vi "SaveasPython.vi"(11 "Graph in":refnum<vi>) -> ()   [LabVIEW 2022 SP3]
uses:
  <vilib>/Utility/error.llb/Trim Whitespace One-Sided.vi
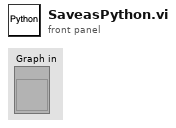
[diagram p1: front panel]
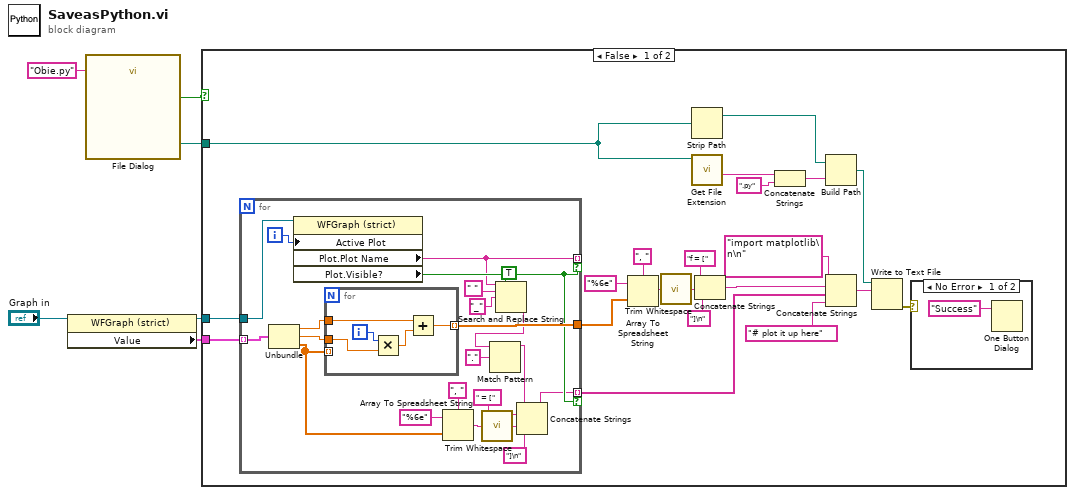
[diagram p0: block diagram]
diagram:
  n1 = property on="Property Node" class="WFGraph (strict)"(reference="Graph in") -> (reference out=w6:refnum<vi>, "Value"=w5:cluster{"x0":dbl, "df":dbl, dbl[]}[])  [unwired: 1 in, 1 out]
  n2 = call "File Dialog"("default name"="Obie.py") -> ("selected path"=w3:path, "cancelled"=w2:bool)  [unwired: 11 in, 2 out]
  n3 = case shown="False" w2 {
    tunnel: w6 -> [w23 _]
    tunnel: w5 -> [w22 _]
    tunnel: w3 -> [w21 _]
    frame False {
      n4 = for {
        tunnel: [w48] -> w13
        tunnel: w22 -> [w47] mode=indexing
        tunnel: [w38] -> w10 mode=indexing if=w44
        tunnel: [w35] -> _ mode=indexing if=w44
        tunnel: w23 -> [w46]
        i -> [w45]
        n5 = Unbundle(w47) -> ("x0"=w49:dbl, "df"=w50:dbl, w42:dbl[])
        n6 = property on="Property Node" class="WFGraph (strict)"(reference=w46, "Active Plot"=w45) -> ("Plot.Plot Name"=w35:string, "Plot.Visible?"=w44:bool)  [unwired: 1 in, 2 out]
        n7 = for {
          tunnel: w50 -> [w54]
          tunnel: w49 -> [w52]
          tunnel: [w51] -> w48 mode=indexing
          tunnel: w42 -> [_] mode=indexing
          i -> [w53]
          n8 = Multiply(x=w53, y=w54) -> (x*y=w55:dbl)
          n9 = Add(x=w52, y=w55) -> (x+y=w51:dbl)
        }
        n10 = Array To Spreadsheet String(delimiter (Tab)=", ", array=w42, 3:"%6e" ("format string")) -> (spreadsheet string=w40:string)
        n11 = call <vilib>:"Trim Whitespace.vi"("string"=w40) -> ("trimmed string"=w36:string)  [unwired: 1 in]
        n12 = Search and Replace String(replace all?=TRUE ("replace all? (F)"), input string=w35, search string=" ", replace string="_" ("replace string (\"\")")) -> (result string=w31:string)  [unwired: 4 in, 3 out]
        n13 = Match Pattern(string=w31, regular expression=".") -> (before substring=w30:string)  [unwired: 1 in, 3 out]
        n14 = Concatenate Strings(w30, " = [" ("delimiter (Tab)"), w36, "]\n" ("string")) -> (w38:string)
      }
      n15 = Array To Spreadsheet String(delimiter (Tab)=", ", array=w13, 3:"%6e" ("format string")) -> (spreadsheet string=w15:string)
      n16 = call <vilib>:"Trim Whitespace.vi"("string"=w15) -> ("trimmed string"=w7:string)  [unwired: 1 in]
      n17 = Strip Path(path=w21) -> (stripped path=w26:path)  [unwired: 1 out]
      n18 = call <vilib>:"Get File Extension.vi"("file"=w21) -> ("filename without extension"=w27:string)  [unwired: 6 in, 4 out]
      n19 = Concatenate Strings("f = [" ("delimiter (Tab)"), w7, "]\n" ("string")) -> (w11:string)
      n20 = Concatenate Strings(w27, ".py" ("string")) -> (w24:string)
      n21 = Build Path(base path=w26, name or relative path=w24) -> (appended path=w19:path)
      n22 = Concatenate Strings("import matplotlib\n\n" ("string"), w11, w10, "# plot it up here" ("string")) -> (w18:string)
      n23 = Write to Text File(file (use dialog)=w19, text=w18) -> (error out=w20:errorcluster)  [unwired: 2 in, 2 out]
      n24 = case shown="No Error" w20 {
        frame No Error {
          n25 = One Button Dialog(message="Success") -> ()  [unwired: 1 in, 1 out]
        }
        frame Error {
        }
      }
    }
    frame True {
    }
  }
